vi "SwerveConfig_Get.vi"() -> (0 "RearRightHome":dbl, 1 "RearLeftHome":dbl, 2 "FrontRightHome":dbl, 3 "FrontLeftHome":dbl)   [LabVIEW 2018]
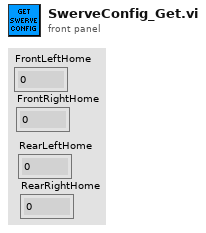
[diagram p1: front panel]
types:
  T1 = enum16{"open", "replace", "create", "open or create", "replace or create", "replace or create with confirmation"}
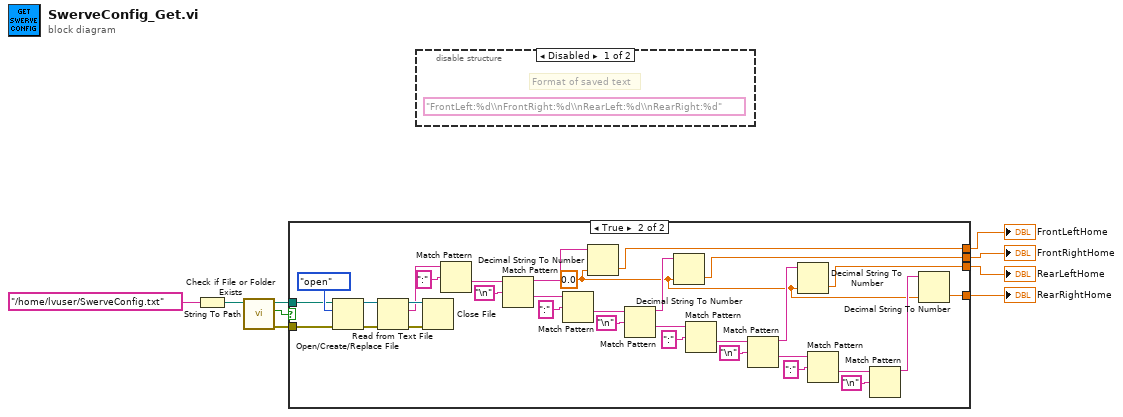
[diagram p0: block diagram]
diagram:
  n1 = String To Path(string="/home/lvuser/SwerveConfig.txt" ("directory path")) -> (path=w8:path)
  n2 = call <vilib>:"Check if File or Folder Exists.vi"("path"=w8) -> ("error out"=w5:errorcluster, "file or folder exists?"=w6:bool, "dup path"=w7:path)  [unwired: 8 in]
  n3 = case shown="True" w6 {
    tunnel: w7 -> [_ w34]
    tunnel: w5 -> [_ w33]
    tunnel: [_ w13] -> w4
    tunnel: [_ w12] -> w3
    tunnel: [_ w11] -> w2
    tunnel: [_ w10] -> w1
    frame False {
      # "File not found, output default:  0"
    }
    frame True {
      w14 = 0.0 ("P")
      n4 = Open/Create/Replace File(file path (use dialog)=w34, error in=w33, operation (0:open)=T1."open") -> (refnum out=w39:refnum<file>, error out=w38:errorcluster)  [unwired: 3 in, 1 out]
      n5 = Read from Text File(file (use dialog)=w39, error in=w38) -> (refnum out=w41:refnum<file>, text=w35:string, error out=w37:errorcluster)  [unwired: 2 in, 1 out]
      n6 = Close File(refnum=w41, error in=w37) -> ()  [unwired: 2 out]
      n7 = Match Pattern(string=w35, regular expression=":") -> (after substring=w31:string)  [unwired: 1 in, 3 out]
      n8 = Match Pattern(string=w31, regular expression="\n") -> (before substring=w18:string, after substring=w21:string)  [unwired: 1 in, 2 out]
      n9 = Match Pattern(string=w21, regular expression=":") -> (after substring=w30:string)  [unwired: 1 in, 3 out]
      n10 = Decimal String To Number(string=w18, default (0L)=w14) -> (number=w13:dbl)  [unwired: 1 in, 1 out]
      n11 = Match Pattern(string=w30, regular expression="\n") -> (before substring=w17:string, after substring=w20:string)  [unwired: 1 in, 2 out]
      n12 = Decimal String To Number(string=w17, default (0L)=w14) -> (number=w12:dbl)  [unwired: 1 in, 1 out]
      n13 = Match Pattern(string=w20, regular expression=":") -> (after substring=w25:string)  [unwired: 1 in, 3 out]
      n14 = Match Pattern(string=w25, regular expression="\n") -> (before substring=w16:string, after substring=w19:string)  [unwired: 1 in, 2 out]
      n15 = Decimal String To Number(string=w16, default (0L)=w14) -> (number=w11:dbl)  [unwired: 1 in, 1 out]
      n16 = Match Pattern(string=w19, regular expression=":") -> (after substring=w24:string)  [unwired: 1 in, 3 out]
      n17 = Match Pattern(string=w24, regular expression="\n") -> (before substring=w15:string)  [unwired: 1 in, 3 out]
      n18 = Decimal String To Number(string=w15, default (0L)=w14) -> (number=w10:dbl)  [unwired: 1 in, 1 out]
    }
  }
  "FrontLeftHome" <- w4
  "FrontRightHome" <- w3
  "RearLeftHome" <- w2
  "RearRightHome" <- w1
  n19 = disable-structure shown="Disabled" {
    frame Disabled {
      (unwired) "FrontLeft:%d\\nFrontRight:%d\\nRearLeft:%d\\nRearRight:%d" ("format string")
      # "Format of saved text"
    }
    frame Enabled {
    }
  }
